vi "Get all axes.vi"(0 "System no.":i32=1 min=1 max=4 step=1) -> (14 "Conn. Axes":string[](array[string]))   [LabVIEW 2020]
doc: "This VI reads all connected axes for given system from Global2 (Array).vi. Connected axes are defined by Define connected axes.vi, which is called by PI_GCS2_Configuration_Setup.vi automatically."
uses:
  Global2 (Array).vi
panel:
  # "This VI returns the defined axes \nfor the given system number."
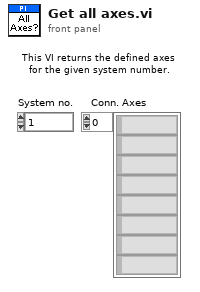
[diagram p1: front panel]
types:
  T1 = typedef "Controller names.ctl" = enum16{"None", "Analog", "C-702", "C-413", "C-414", "C-843", "C-843.PM", "C-844", "C-848", "C-865", "C-866", "C-867", "C-877", "C-880", "C-884", "C-885", "C-886", "C-887", "C-891", "E-135", "E-516", "E-517", "E-518", "E-709", "E-710", "E-712", "E-725", "E-727", "E-753", "E-754", "E-755", "E-761", "E-816", "E-861", "E-870", "E-871", "E-872", "E-873", "E-874", "F-206", "HydraPollux", "M-840", "M-850", "M-8X0", "Mercury", "Mercury_GCS", "PI_GCS2"}
  T2 = cluster{"Conn. axes":string[], "Controller name":T1}[]
  T3 = cluster{"Conn. axes":string[], "Controller name":T1}
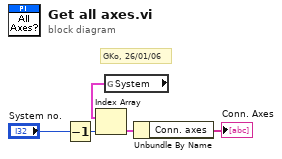
[diagram p0: block diagram]
diagram:
  # "GKo, 26/01/06"
  n1 = Decrement(x="System no.") -> (x-1=w5:i32)
  n2 = global read "Global2 (Array).vi" "System"() -> (w4:T2)
  n3 = Index Array(array=w4, index=w5) -> (element=w2:T3)
  n4 = Unbundle By Name(w2) -> ("Conn. axes"=→"Conn. Axes":string[])
